vi "Create All Message Queues (RT).vi"(8 "error in (no error)":errorcluster) -> (0 "error out":errorcluster, 3 "Message Queues out":T1)   [LabVIEW 2018, in "Message Queue.lvlib"]
doc: "This VI creates and initializes all the message queues for your application. If your application requires more than one message queue, right-click the \"Message Queues\" constant above and select Open Type Def. Add the new Message Queue(s) to the type definition, then initialize them in this VI."
uses:
  Message Queue.lvlib
  All Message Queues (RT).ctl
  Message Cluster (enum).ctl
  Message (enum).ctl
  Message Cluster (string).ctl
  Enqueue Message (string).vi
  Enqueue Message (enum).vi
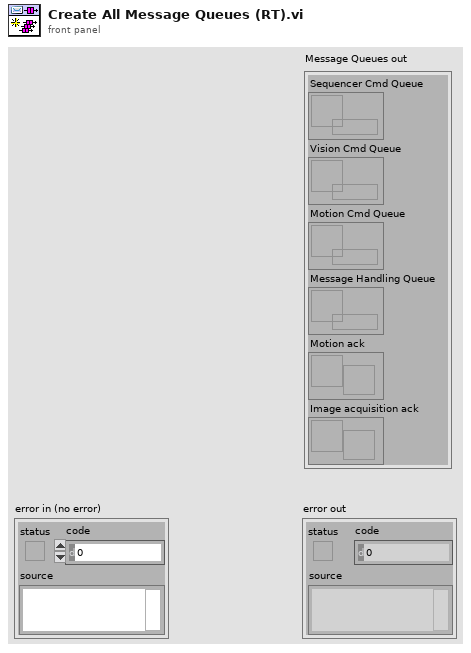
[diagram p1: front panel]
types:
  T1 = typedef "Message Queue.lvlib/All Message Queues (RT).ctl" = cluster{"Sequencer Cmd Queue":refnum<queue>, "Vision Cmd Queue":refnum<queue>, "Motion Cmd Queue":refnum<queue>, "Message Handling Queue":refnum<queue>, "Motion ack":refnum<notifier>, "Image acquisition ack":refnum<notifier>}
  T2 = typedef "Message Queue.lvlib/Message (enum).ctl" = enum16{"Initialize", "Idle", "Running", "Stop", "Pause", "Resume", "Load Sequence File", "Load Sequence from UI", "Save Sequence File"}
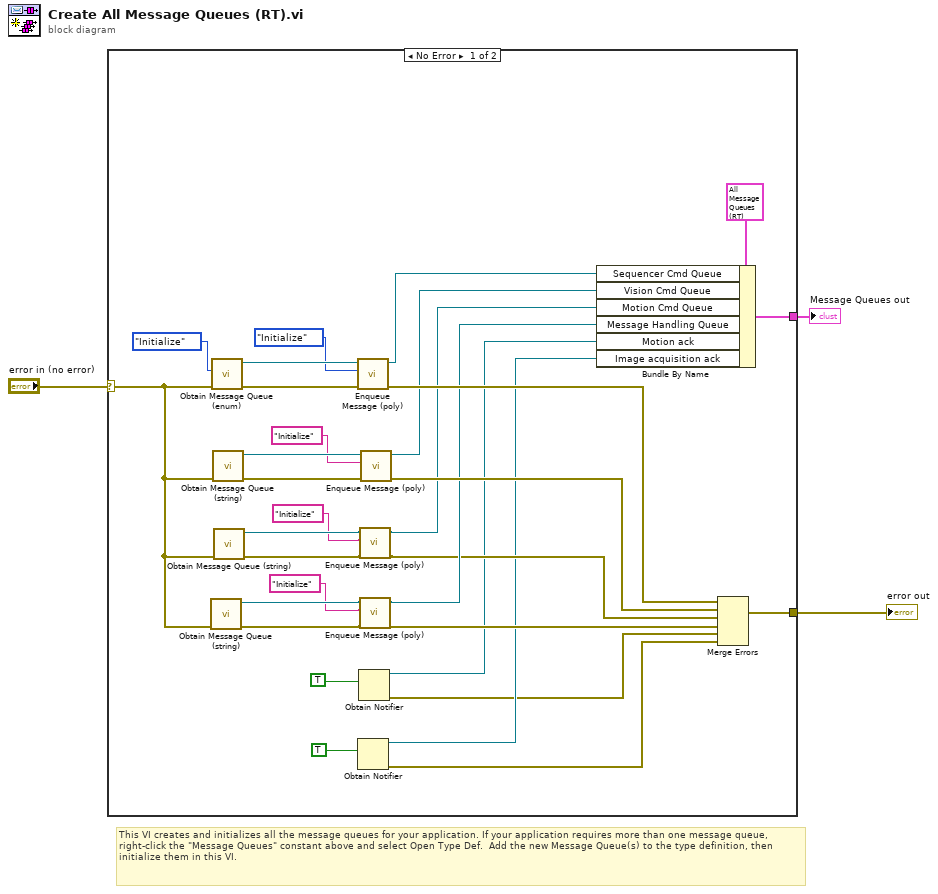
[diagram p0: block diagram]
diagram:
  # "This VI creates and initializes all the message queues for your application. If your application requires more than one message queue, right-click the \"Message Queues\" constant above and select Open Type Def.  Add the new Message Queue(s) to the type definition, then initialize them in this VI."
  n1 = case shown="No Error" "error in (no error)" {
    selector: "error in (no error)" -> [w11 w35]
    tunnel: [w32 w35] -> w3
    tunnel: [w33 _] -> w2
    frame No Error {
      n2 = call "Obtain Message Queue (string).vi"("error in (no error)"=w11) -> ("error out"=w19:errorcluster, "queue out"=w20:refnum<queue>)  [unwired: 9 in]
      n3 = call "Obtain Message Queue (enum).vi"("error in (no error)"=w11, "Message"=Message_(enum)."Initialize" ("Enum")) -> ("error out"=w31:errorcluster, "queue out"=w29:refnum<queue>)  [unwired: 8 in]
      n4 = call "Obtain Message Queue (string).vi"("error in (no error)"=w11) -> ("error out"=w26:errorcluster, "queue out"=w25:refnum<queue>)  [unwired: 9 in]
      n5 = call "Obtain Message Queue (string).vi"("error in (no error)"=w11) -> ("error out"=w15:errorcluster, "queue out"=w23:refnum<queue>)  [unwired: 9 in]
      n6 = call-poly "Enqueue Message (poly).vi"("error in (no error)"=w31, "Enum"=Message_(enum)."Initialize", "Message Queue"=w29) -> ("error out"=w30:errorcluster, "dup Message Queue"=w12:refnum<queue>)  [unwired: 7 in]
      n7 = Obtain Notifier(notification data type=TRUE) -> (notifier out=w9:refnum<notifier>, error out=w7:errorcluster)  [unwired: 3 in, 1 out]
      n8 = Obtain Notifier(notification data type=TRUE) -> (notifier out=w4:refnum<notifier>, error out=w8:errorcluster)  [unwired: 3 in, 1 out]
      n9 = call-poly "Enqueue Message (poly).vi"("error in (no error)"=w15, "Message"="Initialize", "Message Queue"=w23) -> ("error out"=w14:errorcluster, "dup Message Queue"=w22:refnum<queue>)  [unwired: 7 in]
      n10 = call-poly "Enqueue Message (poly).vi"("error in (no error)"=w19, "Message"="Initialize", "Message Queue"=w20) -> ("error out"=w18:errorcluster, "dup Message Queue"=w21:refnum<queue>)  [unwired: 7 in]
      n11 = call-poly "Enqueue Message (poly).vi"("error in (no error)"=w26, "Message"="Initialize", "Message Queue"=w25) -> ("error out"=w27:errorcluster, "dup Message Queue"=w28:refnum<queue>)  [unwired: 7 in]
      n12 = Bundle By Name(cluster=T1 {"Sequencer Cmd Queue"=refnum, "Vision Cmd Queue"=refnum, "Motion Cmd Queue"=refnum, "Message Handling Queue"=refnum, "Motion ack"=refnum, "Image acquisition ack"=refnum} ("Message Queues"), "Sequencer Cmd Queue"=w12, "Vision Cmd Queue"=w28, "Motion Cmd Queue"=w22, "Message Handling Queue"=w21, "Motion ack"=w4, "Image acquisition ack"=w9) -> (w33:T1)
      n13 = Merge Errors(w30, w27, w14, w18, w8, w7) -> (w32:errorcluster)
    }
    frame Error {
    }
  }
  "Message Queues out" <- w2
  "error out" <- w3
